vi "RS-485 Transceiver Control.vi"() -> ()   [LabVIEW 2019]
doc: "This example sets the RS-485 transceiver control modes for the specified port and performs a serial port read, a serial port write, or a combination of these actions. If all are selected, the VI will write the data first, read data and then close the VISA session that is opened to the port. This VI will wait until the specified number of bytes is received at the port or until a termination character is received. This example will work only with National Instruments RS-485 interfaces.\n\nThis example demonstrates the transceiver control modes available when using a National Instruments RS-485 product. When connecting one or several devices via RS-485, a user may want to cut down on the amount of wiring. Alternatively, some devices offer a certain wiring configuration that you may need to match. Determine the wiring needs of the connected serial device to determine which NI RS-485 transceiver control mode to choose.\n\nWhen you are communicating with a two-wire device, National Instruments recommends that you use the two-wire Auto Control mode. This mode handles the transmitter/receiver enabling for a two-wire connection in your hardware, so it reduces the software overhead required to perform this operation in your application program."
uses:
  Program Files (x86)/National Instruments/LabVIEW 2019/examples/Instrument IO/Serial/support/Serial - Settings.ctl
  <vilib>/Instr/_visa.llb/VISA Configure Serial Port (Instr).vi
  <vilib>/Analysis/NI_AALBase.lvlib
panel:
  out "Waveform Chart 2":dynamicdata(graph)
  in  "Count(mSec)":u32
  in  "stop":bool
  out "x*y":dbl
  out "number 4":u32
  out "number 3":u32
  out "number 2":u32
  out "number":u32
  out "element 2":u8
  out "element 3":u8
  out "element 1":u8
  out "Waveform Chart":dbl(graph)
  in  "Termination Character":u8=10 format="%.0x"
  in  "End Write on Termination Character?":bool=TRUE
  in  "End Read on Termination Character?":bool=TRUE
  in  "RS-485 Transceiver Mode":u16(ring) items=["Wire4", "Wire2-EchoDTR", "Wire2-CtrlDTR", "Wire2-Auto"]
  in  "Write String":string="*IDN?"
  in  "Serial Settings":T1={"baud rate"=9600, "data bits"=8, "parity"=enum."None", "stop bits"=10, "flow control"=0} {"flow control" items=["None"=0, "XON/XOFF"=1, "RTS/CTS"=2, "DTR/DSR"=4]; "stop bits" items=["1.0"=10, "1.5"=15, "2.0"=20]; "data bits" min=5 max=8 step=1; "baud rate" items=["75"=75, "110"=110, "134"=134, "150"=150, "300"=300, "600"=600, "1200"=1200, "1800"=1800, "2400"=2400, "4800"=4800, "7200"=7200, "9600"=9600, "14400"=14400, "19200"=19200, "28800"=28800, "38400"=38400, "56000"=56000, "57600"=57600, "115200"=115200, "128000"=128000, "230400"=230400]}
  in  "Assert DTR?":bool
  out "Response":string
  in  "VISA RS 485 Resource":refnum<visa-resource-name>="COM1"
  # "Overview: Demonstrates the use of the VISA functions to configure NI RS-485 hardware.\nRequirements: NI-Serial and NI-VISA Drivers, NI RS-485 hardware\nInstructions:\n1. Ensure the resource specified in the VISA RS 485 Resource control is a valid NI RS-485 device, and that the Assert DTR? value is correct for your device.\n2. Specify the proper RS-485 Transceiver Mode value for your device.\n3. Run the VI.\n4. View the Response returned by the device."
  # "0xA is equivalent to a '\\n' character, which is a line feed."
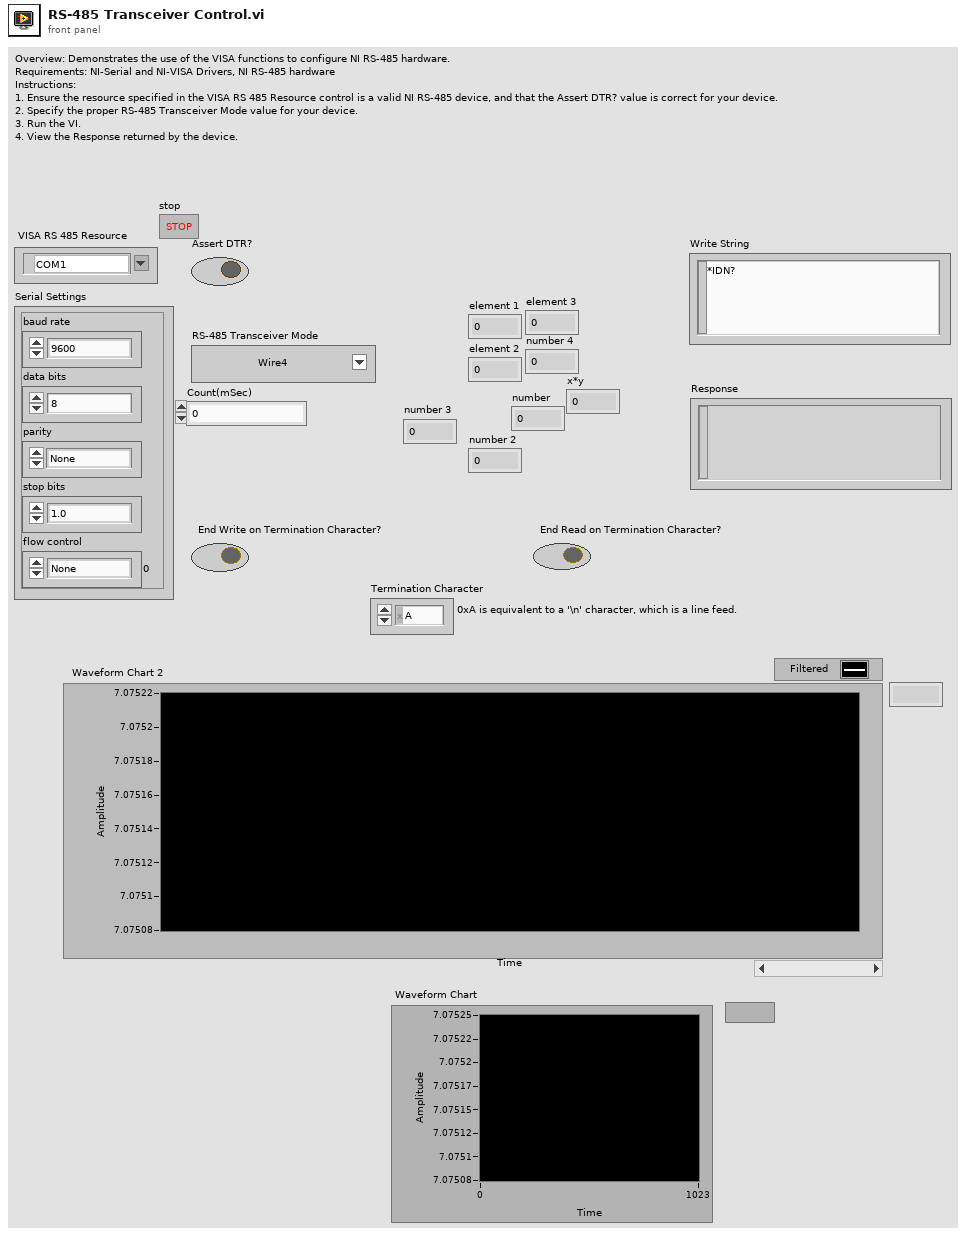
[diagram p1: front panel]
types:
  T1 = typedef "Serial - Settings.ctl" = cluster{"baud rate":u32, "data bits":u16, "parity":enum16{"None", "Odd", "Even", "Mark", "Space"}, "stop bits":u16, "flow control":u16}
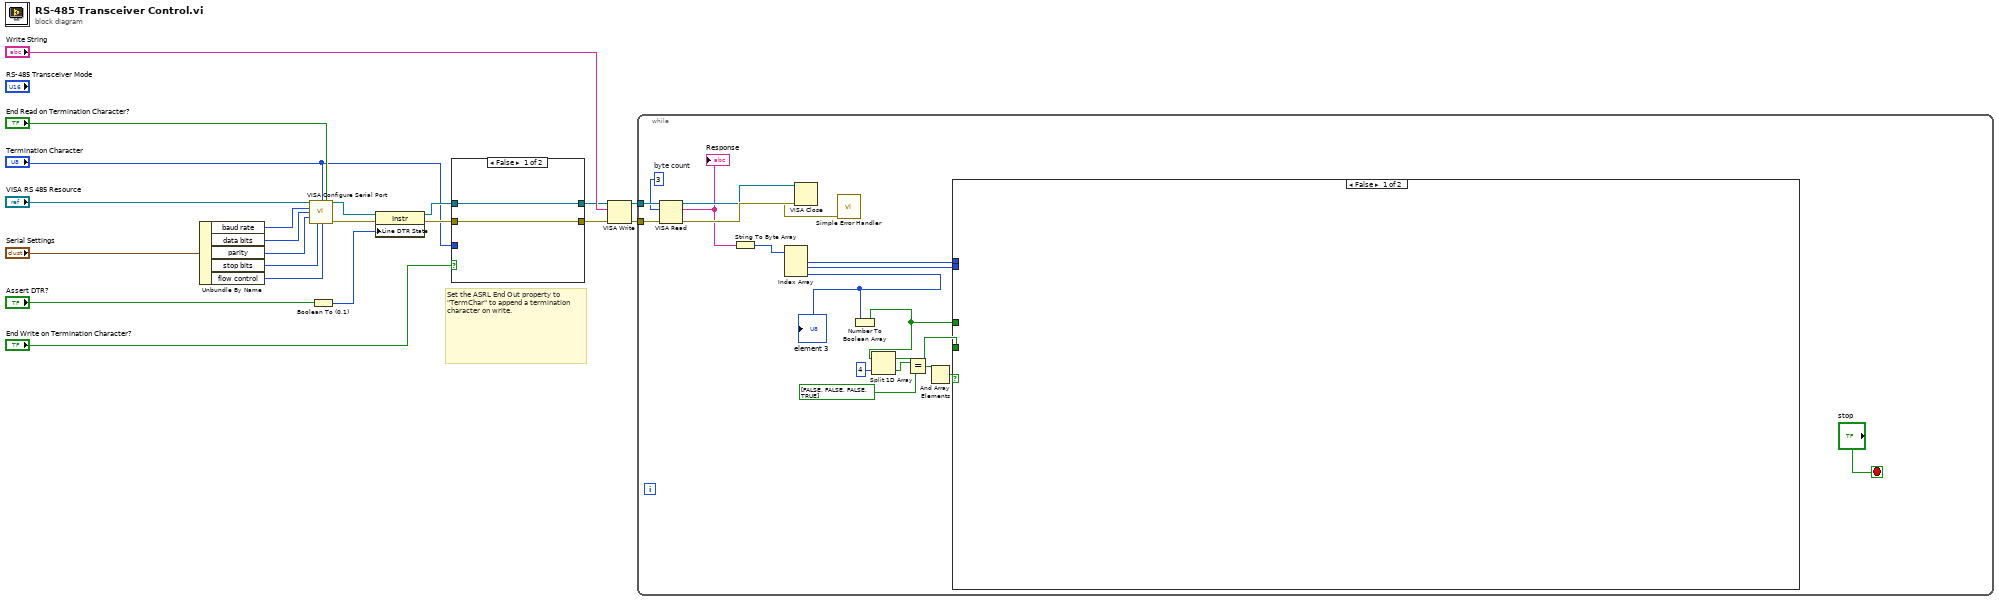
[diagram p0: block diagram]
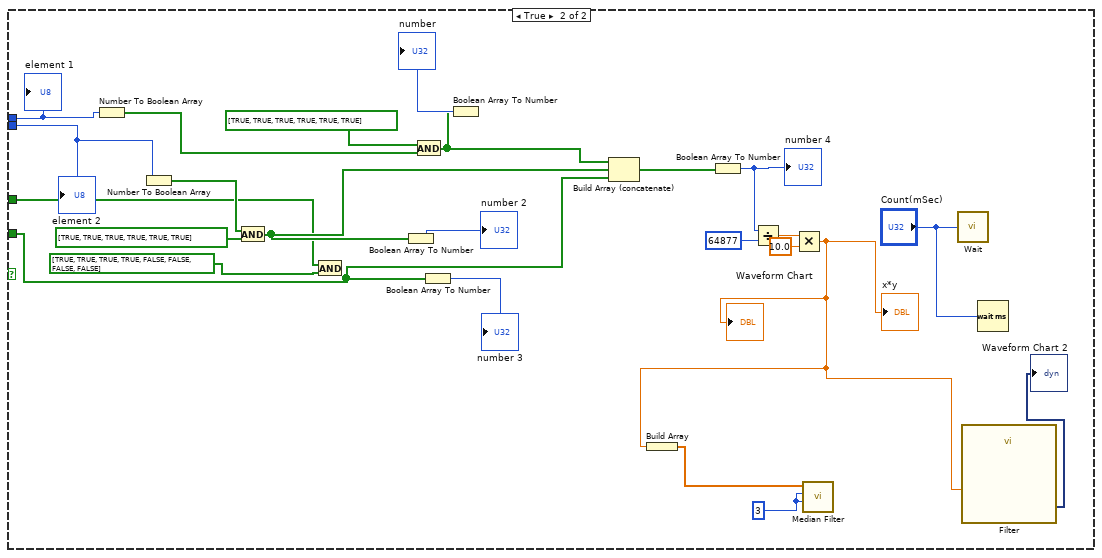
[diagram p2: hidden frame]
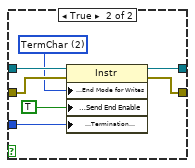
[diagram p3: hidden frame]
diagram:
  # "Set the ASRL End Out property to \"TermChar\" to append a termination character on write."
  n1 = Unbundle By Name("Serial Settings") -> ("baud rate"=w13:u32, "data bits"=w12:u16, "parity"=w11:enum16{"None", "Odd", "Even", "Mark", "Space"}, "stop bits"=w10:u16, "flow control"=w9:u16)
  n2 = call-poly "VISA Configure Serial Port"("VISA resource name"="VISA RS 485 Resource", "termination char\n(0xA = '\\n' = LF)"="Termination Character", "Enable Termination\nChar (T)"="End Read on Termination Character?", "baud rate (921600)"=w13, "data bits (8)"=w12, "parity (0:none)"=w11, "stop bits (10: 1 bit)"=w10, "flow control (0:none)"=w9) -> ("VISA resource name out"=w19:refnum<visa-resource-name>, "error out"=w18:errorcluster)  [unwired: 2 in, 4 out]
  n3 = Boolean To (0,1)(Boolean="Assert DTR?") -> (0, 1=w16:i16)
  n4 = property class="Instr"(reference=w19, error in=w18, "Serial Settings:Modem Line Settings:Line DTR State"=w16) -> (reference out=w4:refnum<visa-resource-name>, error out=w5:errorcluster)
  n5 = case shown="False" "End Write on Termination Character?" {
    tunnel: w4 -> [w22 w30]
    tunnel: w5 -> [w23 w29]
    tunnel: [w22 w28] -> w3
    tunnel: [w23 w27] -> w6
    tunnel: "Termination Character" -> [_ w25]
    frame False {
    }
    frame True {
      w26 = u16 2 items=["None", "LastBit", "TermChar", "Break"] ("Serial Settings:Serial End Mode for Writes")
      n6 = property class="Instr"(reference=w30, error in=w29, "Serial Settings:End Mode for Writes"=w26, "Message Based Settings:Send End Enable"=TRUE, "Message Based Settings:Termination Character"=w25) -> (reference out=w28:refnum<visa-resource-name>, error out=w27:errorcluster)
    }
  }
  n7 = VISA Write(VISA resource name=w3, write buffer="Write String", error in (no error)=w6) -> (VISA resource name out=w20:refnum<visa-resource-name>, error out=w15:errorcluster)  [unwired: 1 out]
  n8 = while {
    tunnel: w20 -> [w49]
    tunnel: w15 -> [w46]
    stop <- "stop" stop-if-true
    w44 = u32 3  # byte count
    n9 = VISA Read(VISA resource name=w49, byte count=w44, error in (no error)=w46) -> (VISA resource name out=w47:refnum<visa-resource-name>, read buffer=w43:string, error out=w48:errorcluster)  [unwired: 1 out]
    "Response" <- w43
    n10 = String To Byte Array(string=w43) -> (unsigned byte array=w42:u8[])
    n11 = Index Array(array=w42) -> (element #1=w41:u8, element #2=w40:u8, element #3=w39:u8)  [unwired: 3 in]
    "element 3" <- w39
    n12 = VISA Close(VISA resource name=w47, error in (no error)=w48) -> (error out=w45:errorcluster)
    n13 = call <vilib>:"Simple Error Handler.vi"("error in (no error)"=w45) -> ()  [unwired: 1 in, 8 out]
    n14 = Number To Boolean Array(number=w39) -> (Boolean array=w37:bool[])
    n15 = Split 1D Array(array=w37, index=4) -> (first subarray=w31:bool[], second subarray=w32:bool[])
    n16 = Equal?(x=w32, y=bool[] [FALSE, FALSE, FALSE, TRUE]) -> (x = y?=w33:bool[])
    n17 = And Array Elements(Boolean array=w33) -> (logical AND=w34:bool)
    n18 = case shown="False" w34 {
      tunnel: w41 -> [_ w73]
      tunnel: w40 -> [_ w70]
      tunnel: w37 -> [_ w55]
      tunnel: w31 -> [_ w54]
      frame False {
      }
      frame True {
        w52 = 3 ("left rank")
        n19 = Number To Boolean Array(number=w73) -> (Boolean array=w57:bool[])
        n20 = Number To Boolean Array(number=w70) -> (Boolean array=w69:bool[])
        n21 = And(x=w69, y=bool[] [TRUE, TRUE, TRUE, TRUE, TRUE, TRUE] ("x")) -> (x .and. y?=w59:bool[])
        n22 = And(x=w55, y=bool[] [TRUE, TRUE, TRUE, TRUE, FALSE, FALSE, FALSE, FALSE] ("x")) -> ()  [unwired: 1 out]
        n23 = Boolean Array To Number(Boolean array=w59) -> (number=→"number 2":u32)
        n24 = And(x=bool[] [TRUE, TRUE, TRUE, TRUE, TRUE, TRUE], y=w57) -> (x .and. y?=w58:bool[])
        n25 = Boolean Array To Number(Boolean array=w54) -> (number=→"number 3":u32)
        n26 = Boolean Array To Number(Boolean array=w58) -> (number=→"number":u32)
        n27 = Build Array (concatenate)(w58, w59, w54) -> (w64:bool[])
        n28 = Boolean Array To Number(Boolean array=w64) -> (number=w63:u32)
        "number 4" <- w63
        n29 = Divide(x=w63, y=u32 64877) -> (x/y=w61:dbl)
        n30 = Multiply(x=w61, y=10.0) -> (x*y=w51:dbl)
        "Waveform Chart" <- w51
        "x*y" <- w51
        n31 = Build Array(w51) -> (w53:dbl[])
        n32 = call <vilib>:"Median Filter.vi"("right rank"=w52, "left rank"=w52, "X"=w53) -> ()  [unwired: 7 in, 2 out]
        n33 = call "Wait"("Count(mSec)"="Count(mSec)") -> ()  [unwired: 1 out]
        n34 = call "Filter"("Signal"=w51) -> ("Filtered Signal"=→"Waveform Chart 2":dynamicdata)  [unwired: 9 in, 1 out]
        n35 = Wait (ms)(milliseconds to wait="Count(mSec)") -> ()  [unwired: 1 out]
        "element 1" <- w73
        "element 2" <- w70
      }
    }
  }
